vi "Obtain Session.vi"(8 "error in (no error)":errorcluster, 11 "Session  Name ()":string="_default_registry") -> (0 "error out":errorcluster, 3 "Session Handle":T1)   [LabVIEW 2020, in "Registry.lvlib" / "Registry Session.lvclass"]
doc: "Obtains a reference to the registry pointed by its name. Please make sure you close this session with Release Session once you are done interacting with the registry."
uses:
  Registry Session.lvclass
  Typedefs/Session Handle.ctl
  C:/Program Files (x86)/National Instruments/LabVIEW 2020/user.lib/_Session Fwk/Session - Root.lvclass
  <userlib>/_Session Fwk/Session - Root.lvclass
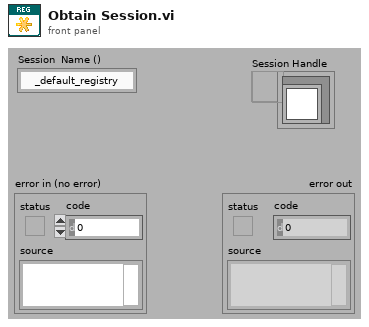
[diagram p1: front panel]
types:
  T1 = typedef "Registry.lvlib/Registry Session.lvclass/Session Handle.ctl" = refnum<data-value>
  T2 = typedef "Session - Root.lvclass/Session Handle.ctl" = refnum<data-value>
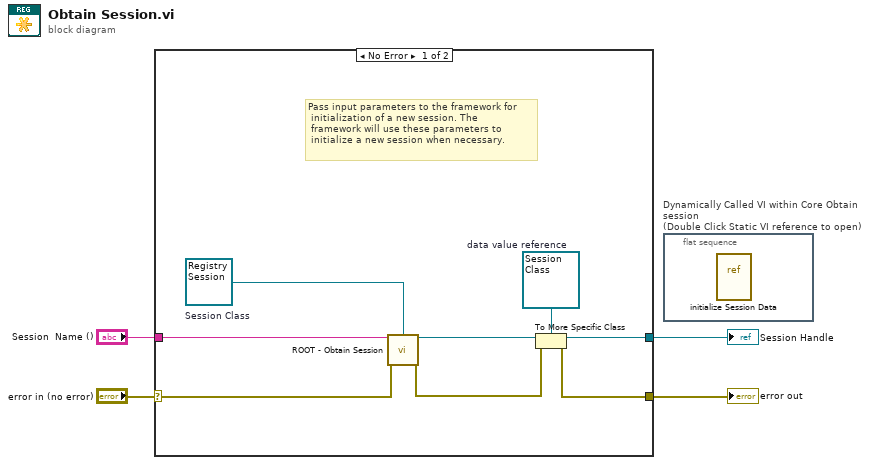
[diagram p0: block diagram]
diagram:
  n1 = case shown="No Error" "error in (no error)" {
    selector: "error in (no error)" -> [w11 w13]
    tunnel: [w8 w13] -> w3
    tunnel: [w10 _] -> w1
    tunnel: "Session  Name ()" -> [w12 _]
    frame No Error {
      w5 = refnum<data-value> refnum  # data value reference
      w6 = refnum<class "Registry Session.lvclass"> refnum  # Session Class
      # "Pass input parameters to the framework for\n initialization of a new session. The\n framework will use these parameters to\n initialize a new session when necessary."
      n2 = call <userlib>:"ROOT - Obtain Session.vi"("Session Name ()"=w12, "OBJ - Session"=w6, "error in (no error)"=w11) -> ("Session Handle"=w7:T2, "error out"=w9:errorcluster)  [unwired: 10 in, 1 out]
      n3 = To More Specific Class(target class=w5, reference=w7, error in=w9) -> (specific class reference=w10:refnum<data-value>, error out=w8:errorcluster)
    }
    frame Error {
    }
  }
  "error out" <- w3
  "Session Handle" <- w1
  n4 = flat-sequence "Dynamically Called VI within Core Obtain session\n(Double Click Static VI reference to open)" {
    frame #0 {
      n5 = vi-ref "initialize Session Data.vi"() -> ()  [unwired: 1 out]
    }
  }
